vi "Step_Forward.vi"(3 "error in":errorcluster, 4 "Data in":T1, 5 "Step control reference in":refnum<vi>) -> (0 "error out":errorcluster, 1 "Data out":T1, 2 "Step control reference out":refnum<vi>)   [LabVIEW 2017]
uses:
  Type_Defs/Data.ctl
  Type_Defs/Diagnostics.ctl
  Type_Defs/Systems.ctl
  Step_Vis/Steps.lvlib
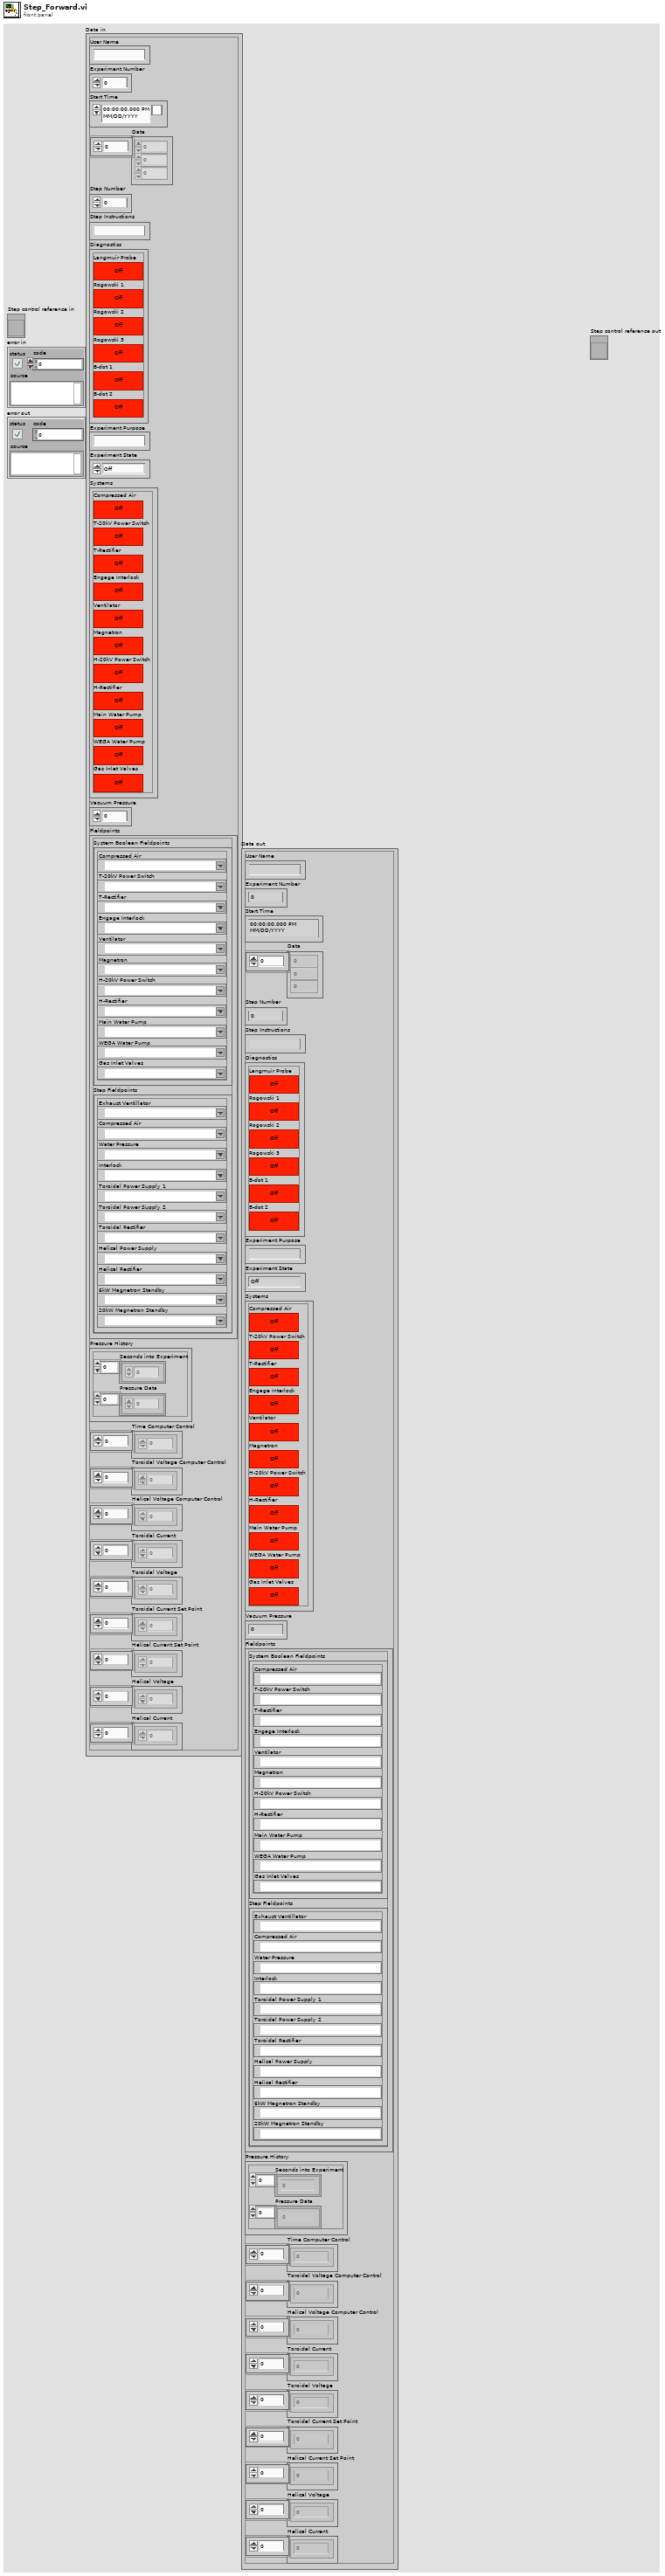
[diagram p1: front panel]
types:
  T1 = typedef "Data.ctl" = cluster{"User Name":string, "Experiment Number":i32, "Start Time":timestamp, "Data":dbl[], "Step Number":i32, "Step Instructions":string, "Diagnostics":T2, "Experiment Purpose":string, "Experiment State":enum16{"Off", "Setting Up", "Ready", "In Progress", "Shutting Down"}, "Systems":T3, "Vacuum Pressure":dbl, "Fieldpoints":cluster{"System Boolean Fieldpoints":cluster{"Compressed Air":refnum<k21>, "T-20kV Power Switch":refnum<k21>, "T-Rectifier":refnum<k21>, "Engage Interlock":refnum<k21>, "Ventilator":refnum<k21>, "Magnetron":refnum<k21>, "H-20kV Power Switch":refnum<k21>, "H-Rectifier":refnum<k21>, "Main Water Pump":refnum<k21>, "WEGA Water Pump":refnum<k21>, "Gas Inlet Valves":refnum<k21>}, "Step Fieldpoints":cluster{"Exhaust Ventillator":refnum<k21>, "Compressed Air":refnum<k21>, "Water Pressure":refnum<k21>, "Interlock":refnum<k21>, "Toroidal Power Supply 1":refnum<k21>, "Toroidal Power Supply 2":refnum<k21>, "Toroidal Rectifier":refnum<k21>, "Helical Power Supply":refnum<k21>, "Helical Rectifier":refnum<k21>, "6kW Magnetron Standby":refnum<k21>, "20kW Magnetron Standby":refnum<k21>}}, "Pressure History":cluster{"Seconds into Experiment":i32[], "Pressure Data":dbl[]}, "Time Computer Control":dbl[], "Toroidal Voltage Computer Control":dbl[], "Helical Voltage Computer Control":dbl[], "Toroidal Current":dbl[], "Toroidal Voltage":dbl[], "Toroidal Current Set Point":dbl[], "Helical Current Set Point":dbl[], "Helical Voltage":dbl[], "Helical Current":dbl[]}
  T2 = typedef "Diagnostics.ctl" = cluster{"Langmuir Probe":bool, "Rogowski 1":bool, "Rogowski 2":bool, "Rogowski 3":bool, "B-dot 1":bool, "B-dot 2":bool}
  T3 = typedef "Systems.ctl" = cluster{"Compressed Air":bool, "T-20kV Power Switch":bool, "T-Rectifier":bool, "Engage Interlock":bool, "Ventilator":bool, "Magnetron":bool, "H-20kV Power Switch":bool, "H-Rectifier":bool, "Main Water Pump":bool, "WEGA Water Pump":bool, "Gas Inlet Valves":bool}
  T4 = enum16{"Off", "Setting Up", "Ready", "In Progress", "Shutting Down"}
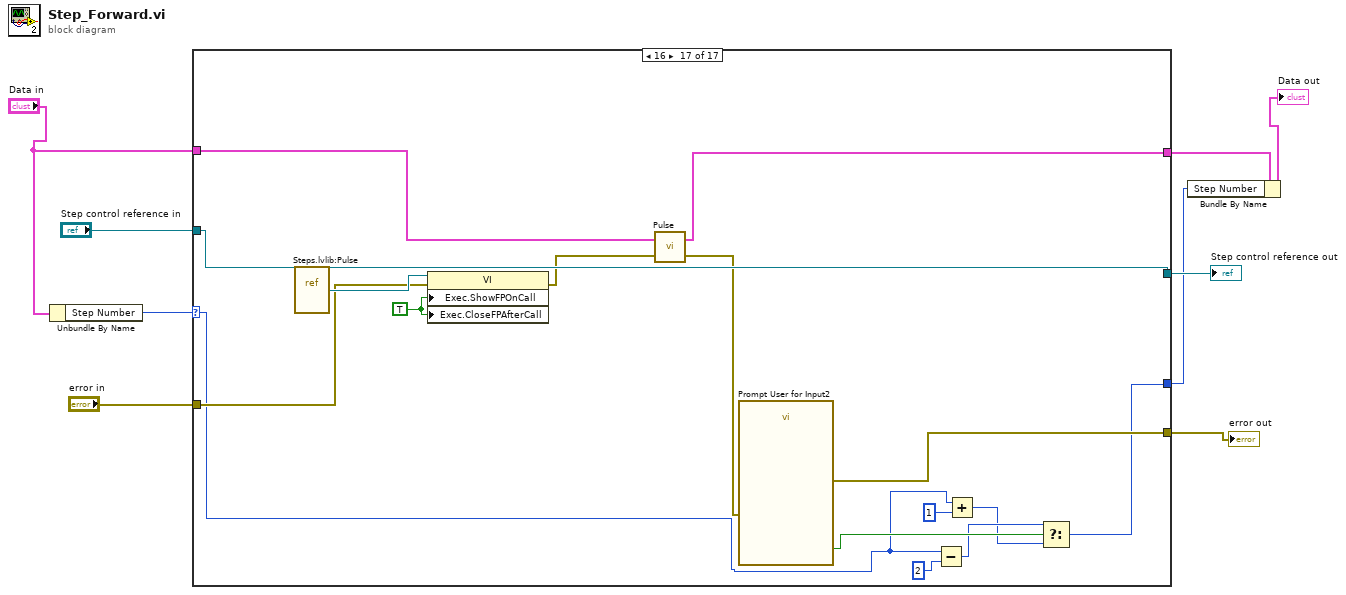
[diagram p0: block diagram]
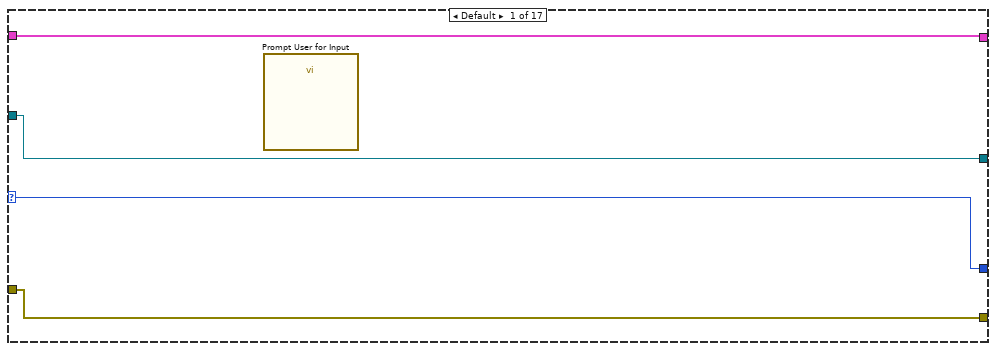
[diagram p2: hidden frame]
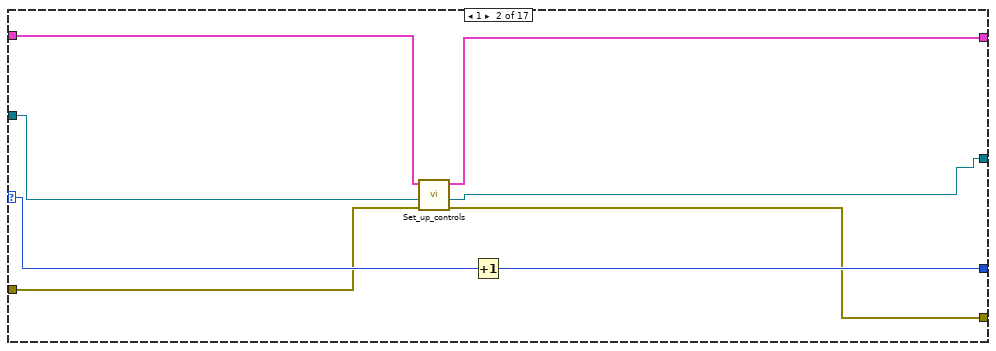
[diagram p3: hidden frame]
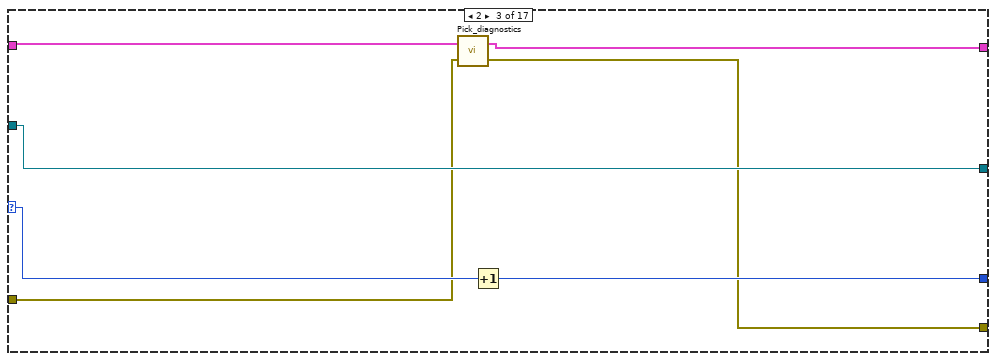
[diagram p4: hidden frame]
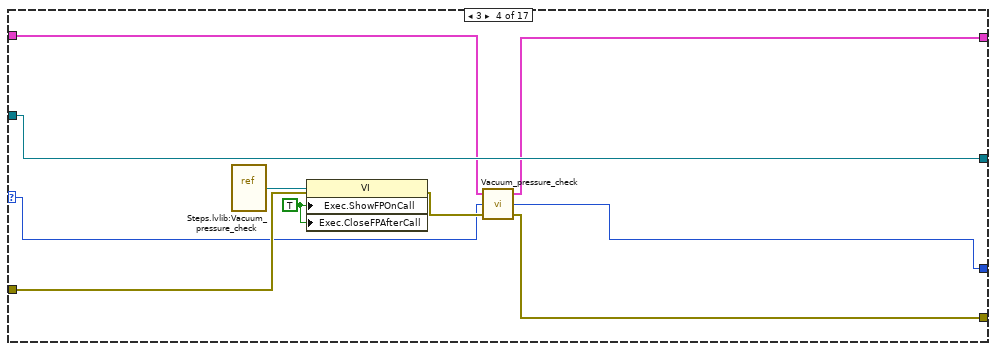
[diagram p5: hidden frame]
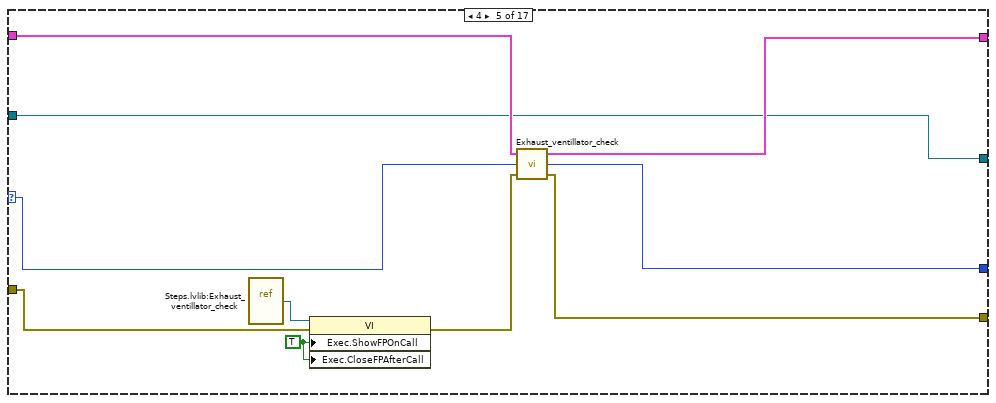
[diagram p6: hidden frame]
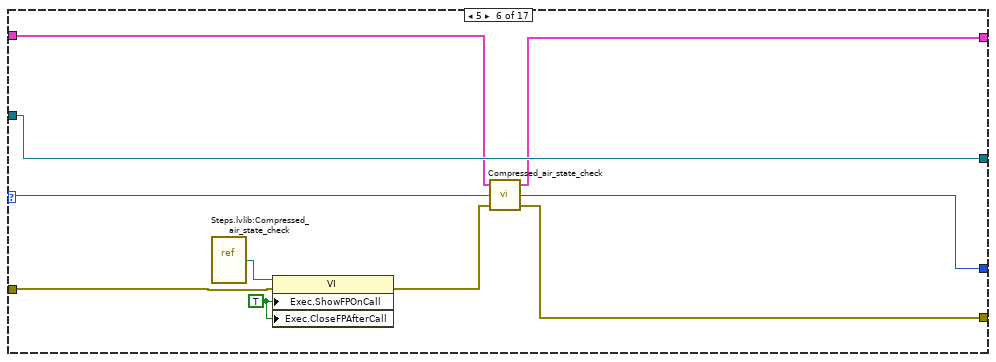
[diagram p7: hidden frame]
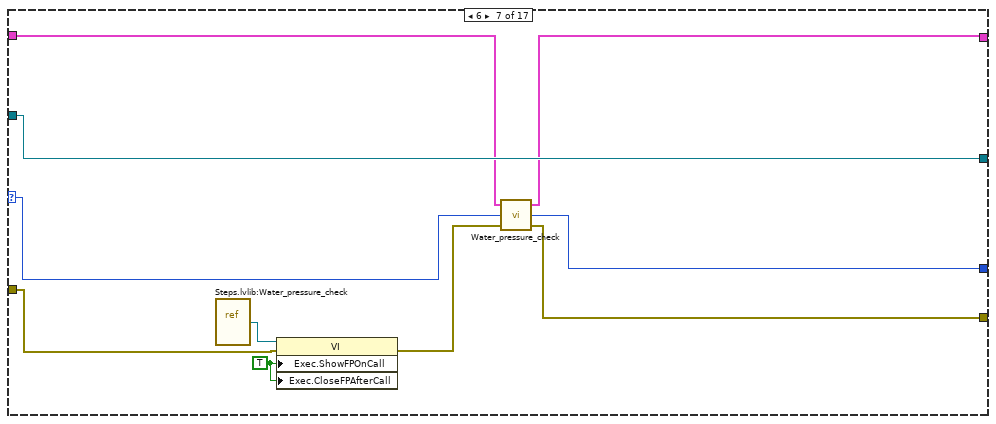
[diagram p8: hidden frame]
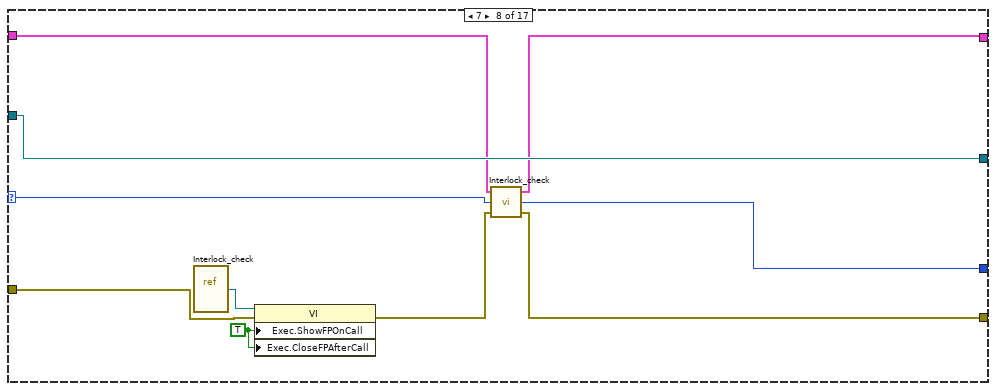
[diagram p9: hidden frame]
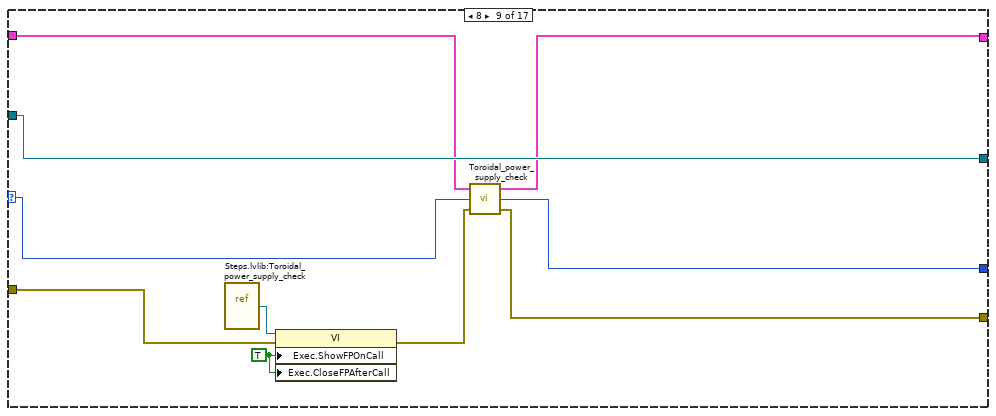
[diagram p10: hidden frame]
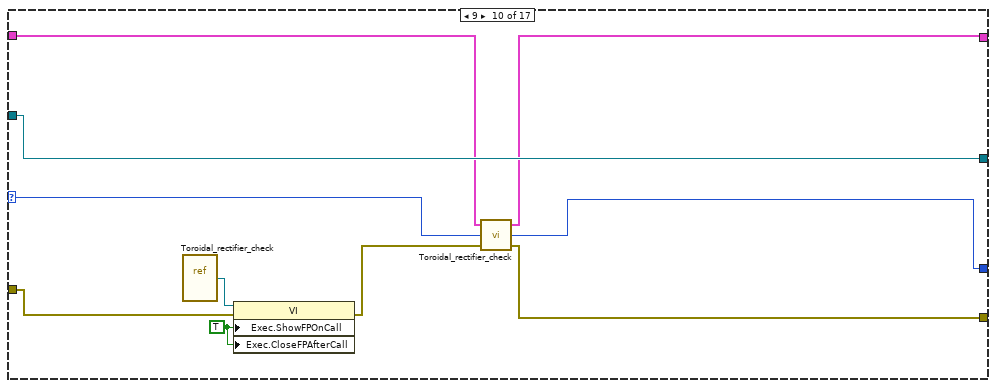
[diagram p11: hidden frame]
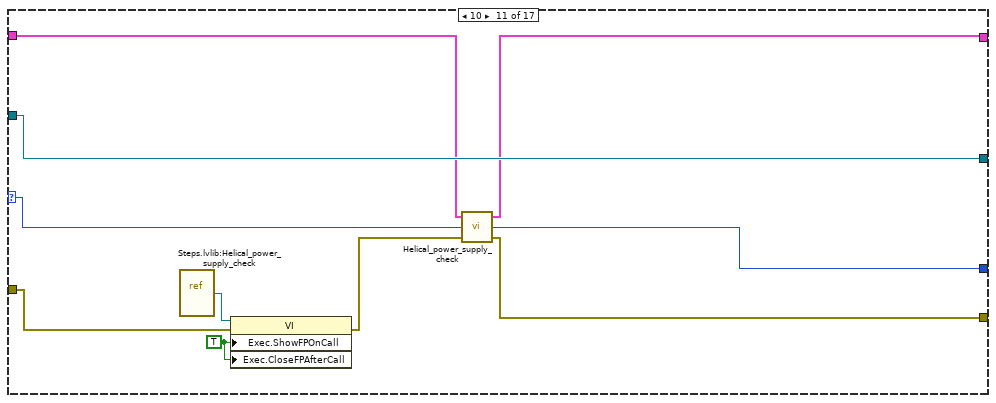
[diagram p12: hidden frame]
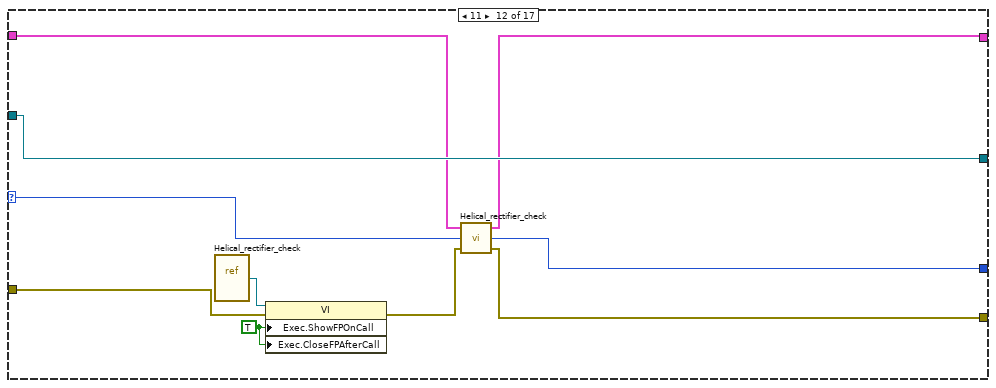
[diagram p13: hidden frame]
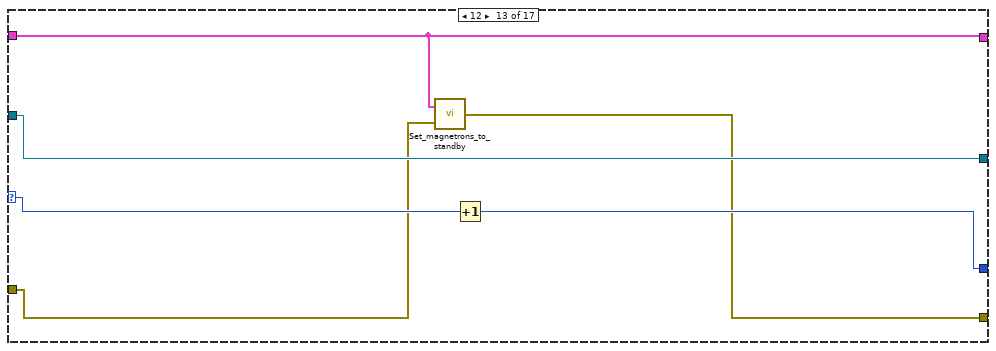
[diagram p14: hidden frame]
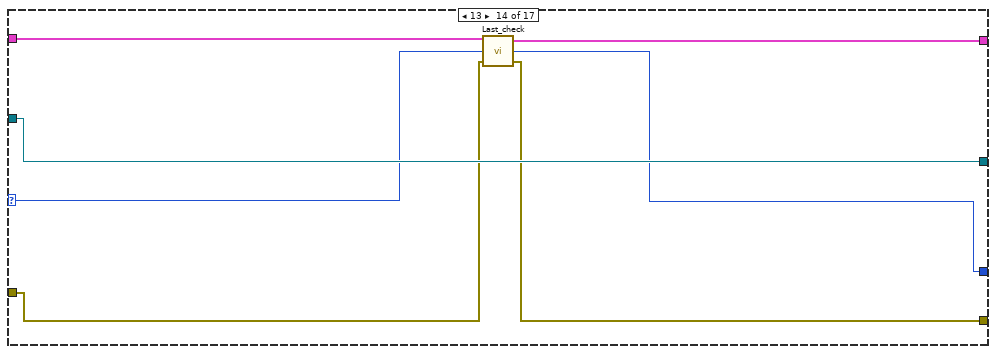
[diagram p15: hidden frame]
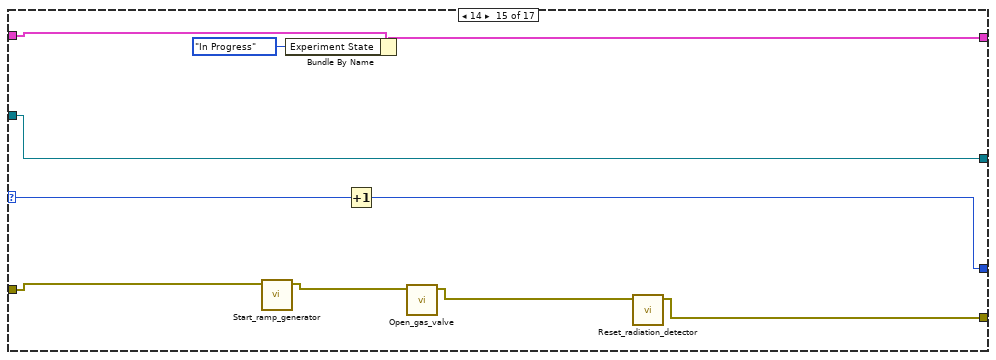
[diagram p16: hidden frame]
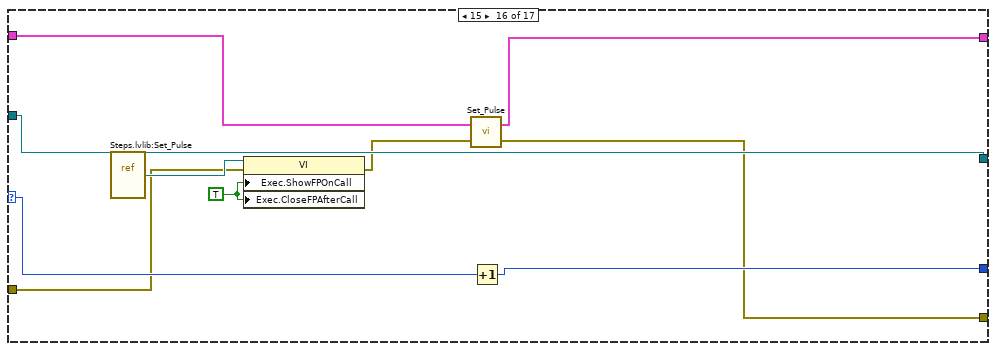
[diagram p17: hidden frame]
diagram:
  n1 = Unbundle By Name("Data in") -> ("Step Number"=w5:i32)
  n2 = case shown="16" w5 {
    selector: w5 -> [w12 w21 w28 w29 w45 w57 w65 w73 w85 w91 w102 w113 w122 w128 w139 w149 w154]
    tunnel: "Step control reference in" -> [w13 w17 w26 w38 w44 w58 w68 w78 w88 w98 w108 w118 w124 w131 w141 w151 w167]
    tunnel: [w13 w14 w26 w38 w44 w58 w68 w78 w88 w98 w108 w118 w124 w131 w141 w151 w167] -> w8
    tunnel: [w12 w20 w27 w30 w46 w53 w64 w74 w84 w92 w101 w112 w123 w127 w140 w150 w155] -> w3
    tunnel: "error in" -> [w11 w19 w25 w36 w41 w49 w59 w69 w82 w95 w105 w109 w120 w126 w138 w144 w162]
    tunnel: [w11 w18 w24 w34 w43 w54 w63 w75 w80 w93 w103 w111 w119 w125 w135 w142 w157] -> w6
    tunnel: "Data in" -> [w10 w16 w23 w32 w48 w55 w67 w77 w87 w90 w100 w115 w121 w130 w134 w146 w164]
    tunnel: [w10 w15 w22 w31 w47 w56 w66 w76 w86 w89 w99 w114 w121 w129 w133 w145 w163] -> w4
    frame Default {
      n3 = call "Prompt User for Input"() -> ()  [unwired: 18 in, 2 out]
    }
    frame 1 {
      n4 = call "Set_up_controls.vi"("error in"=w19, "reference"=w17, "Data in"=w16) -> ("error out"=w18:errorcluster, "reference out"=w14:refnum<vi>, "Data out"=w15:T1)  [unwired: 1 in, 1 out]
      n5 = Increment(x=w21) -> (x+1=w20:i32)
    }
    frame 2 {
      n6 = call "Pick_diagnostics.vi"("error in (no error)"=w25, "Data In"=w23) -> ("error out"=w24:errorcluster, "Data Out"=w22:T1)
      n7 = Increment(x=w28) -> (x+1=w27:i32)
    }
    frame 3 {
      w33 = TRUE ("Execution:Show Front Panel On Call")
      n8 = vi-ref "Steps.lvlib:Vacuum_pressure_check.vi"() -> (w37:refnum<vi>)
      n9 = property class="VI"(reference=w37, error in=w36, "Exec.ShowFPOnCall"=w33, "Exec.CloseFPAfterCall"=w33) -> (error out=w35:errorcluster)  [unwired: 1 out]
      n10 = call "Vacuum_pressure_check.vi"("error in"=w35, "Step Number in"=w29, "Data in"=w32) -> ("error out"=w34:errorcluster, "Step Number out"=w30:i32, "Data out"=w31:T1)
    }
    frame 4 {
      w42 = TRUE ("Execution:Show Front Panel On Call")
      n11 = vi-ref "Steps.lvlib:Exhaust_ventillator_check.vi"() -> (w39:refnum<vi>)
      n12 = property class="VI"(reference=w39, error in=w41, "Exec.ShowFPOnCall"=w42, "Exec.CloseFPAfterCall"=w42) -> (error out=w40:errorcluster)  [unwired: 1 out]
      n13 = call "Exhaust_ventillator_check.vi"("error in"=w40, "Step Number in"=w45, "Data in"=w48) -> ("error out"=w43:errorcluster, "Step Number out"=w46:i32, "Data out"=w47:T1)
    }
    frame 5 {
      w52 = TRUE ("Execution:Show Front Panel On Call")
      n14 = vi-ref "Steps.lvlib:Compressed_air_state_check.vi"() -> (w51:refnum<vi>)
      n15 = property class="VI"(reference=w51, error in=w49, "Exec.ShowFPOnCall"=w52, "Exec.CloseFPAfterCall"=w52) -> (error out=w50:errorcluster)  [unwired: 1 out]
      n16 = call "Compressed_air_state_check.vi"("error in"=w50, "Step Number in"=w57, "Data in"=w55) -> ("error out"=w54:errorcluster, "Step Number out"=w53:i32, "Data out"=w56:T1)
    }
    frame 6 {
      w62 = TRUE ("Execution:Show Front Panel On Call")
      n17 = vi-ref "Steps.lvlib:Water_pressure_check.vi"() -> (w61:refnum<vi>)
      n18 = property class="VI"(reference=w61, error in=w59, "Exec.ShowFPOnCall"=w62, "Exec.CloseFPAfterCall"=w62) -> (error out=w60:errorcluster)  [unwired: 1 out]
      n19 = call "Water_pressure_check.vi"("error in"=w60, "Step Number in"=w65, "Data in"=w67) -> ("error out"=w63:errorcluster, "Step Number out"=w64:i32, "Data out"=w66:T1)
    }
    frame 7 {
      w71 = TRUE ("Execution:Show Front Panel On Call")
      n20 = vi-ref "Interlock_check.vi"() -> (w72:refnum<vi>)
      n21 = property class="VI"(reference=w72, error in=w69, "Exec.ShowFPOnCall"=w71, "Exec.CloseFPAfterCall"=w71) -> (error out=w70:errorcluster)  [unwired: 1 out]
      n22 = call "Interlock_check.vi"("error in"=w70, "Step Number in"=w73, "Data in"=w77) -> ("error out"=w75:errorcluster, "Step Number out"=w74:i32, "Data out"=w76:T1)
    }
    frame 8 {
      w83 = TRUE ("Execution:Show Front Panel On Call")
      n23 = vi-ref "Steps.lvlib:Toroidal_power_supply_check.vi"() -> (w79:refnum<vi>)
      n24 = property class="VI"(reference=w79, error in=w82, "Exec.ShowFPOnCall"=w83, "Exec.CloseFPAfterCall"=w83) -> (error out=w81:errorcluster)  [unwired: 1 out]
      n25 = call "Toroidal_power_supply_check.vi"("error in"=w81, "Step Number in"=w85, "Data in"=w87) -> ("error out"=w80:errorcluster, "Step Number out"=w84:i32, "Data out"=w86:T1)
    }
    frame 9 {
      w97 = TRUE ("Execution:Show Front Panel On Call")
      n26 = vi-ref "Toroidal_rectifier_check.vi"() -> (w96:refnum<vi>)
      n27 = property class="VI"(reference=w96, error in=w95, "Exec.ShowFPOnCall"=w97, "Exec.CloseFPAfterCall"=w97) -> (error out=w94:errorcluster)  [unwired: 1 out]
      n28 = call "Toroidal_rectifier_check.vi"("error in"=w94, "Step Number in"=w91, "Data in"=w90) -> ("error out"=w93:errorcluster, "Step Number out"=w92:i32, "Data out"=w89:T1)
    }
    frame 10 {
      w106 = TRUE ("Execution:Show Front Panel On Call")
      n29 = vi-ref "Steps.lvlib:Helical_power_supply_check.vi"() -> (w107:refnum<vi>)
      n30 = property class="VI"(reference=w107, error in=w105, "Exec.ShowFPOnCall"=w106, "Exec.CloseFPAfterCall"=w106) -> (error out=w104:errorcluster)  [unwired: 1 out]
      n31 = call "Helical_power_supply_check.vi"("error in"=w104, "Step Number in"=w102, "Data in"=w100) -> ("error out"=w103:errorcluster, "Step Number out"=w101:i32, "Data out"=w99:T1)
    }
    frame 11 {
      w116 = TRUE ("Execution:Show Front Panel On Call")
      n32 = vi-ref "Helical_rectifier_check.vi"() -> (w117:refnum<vi>)
      n33 = property class="VI"(reference=w117, error in=w109, "Exec.ShowFPOnCall"=w116, "Exec.CloseFPAfterCall"=w116) -> (error out=w110:errorcluster)  [unwired: 1 out]
      n34 = call "Helical_rectifier_check.vi"("error in"=w110, "Step Number in"=w113, "Data in"=w115) -> ("error out"=w111:errorcluster, "Step Number out"=w112:i32, "Data out"=w114:T1)
    }
    frame 12 {
      n35 = call "Set_magnetrons_to_standby.vi"("error in"=w120, "Data in"=w121) -> ("error out"=w119:errorcluster)
      n36 = Increment(x=w122) -> (x+1=w123:i32)
    }
    frame 13 {
      n37 = call "Last_check.vi"("error in"=w126, "Step Number in"=w128, "Data in"=w130) -> ("error out"=w125:errorcluster, "Step Number out"=w127:i32, "Data out"=w129:T1)
    }
    frame 14 {
      n38 = call "Start_ramp_generator.vi"("error in"=w138) -> ("error out"=w137:errorcluster)  [unwired: 10 in]
      n39 = Bundle By Name(cluster=w134, "Experiment State"=T4."In Progress") -> (w133:T1)
      n40 = Increment(x=w139) -> (x+1=w140:i32)
      n41 = call "Open_gas_valve.vi"("error in"=w137) -> ("error out"=w136:errorcluster)  [unwired: 10 in]
      n42 = call "Reset_radiation_detector.vi"("error in"=w136) -> ("error out"=w135:errorcluster)  [unwired: 10 in]
    }
    frame 15 {
      w148 = TRUE ("Execution:Show Front Panel On Call")
      n43 = vi-ref "Steps.lvlib:Set_Pulse.vi"() -> (w147:refnum<vi>)
      n44 = property class="VI"(reference=w147, error in=w144, "Exec.ShowFPOnCall"=w148, "Exec.CloseFPAfterCall"=w148) -> (error out=w143:errorcluster)  [unwired: 1 out]
      n45 = call "Set_Pulse.vi"("error in"=w143, "Data in"=w146) -> ("error out"=w142:errorcluster, "Data out"=w145:T1)
      n46 = Increment(x=w149) -> (x+1=w150:i32)
    }
    frame 16 {
      w166 = TRUE ("Execution:Show Front Panel On Call")
      n47 = vi-ref "Steps.lvlib:Pulse.vi"() -> (w165:refnum<vi>)
      n48 = property class="VI"(reference=w165, error in=w162, "Exec.ShowFPOnCall"=w166, "Exec.CloseFPAfterCall"=w166) -> (error out=w161:errorcluster)  [unwired: 1 out]
      n49 = call "Pulse.vi"("error in"=w161, "Data in"=w164) -> ("error out"=w158:errorcluster, "Data out"=w163:T1)
      n50 = call "Prompt User for Input2"("error in (no error)"=w158) -> ("Run New Shot"=w160:bool, "error out"=w157:errorcluster)  [unwired: 16 in, 1 out]
      n51 = Subtract(x=w154, y=2) -> (x-y=w153:i32)
      n52 = Add(x=w154, y=1) -> (x+y=w152:i32)
      n53 = Select(t=w153, s=w160, f=w152) -> (s? t:f=w155:i32)
    }
  }
  "Step control reference out" <- w8
  "error out" <- w6
  n54 = Bundle By Name(cluster=w4, "Step Number"=w3) -> (→"Data out":T1)
